vi "User_Event.vi"(0 "Event Data":T1, 11 "Error In":errorcluster, 13 "Enum":T2) -> (4 "Ref Out":refnum<user-event>, 15 "Error Out":errorcluster)   [LabVIEW 2020]
doc: "This VI is used to create, generate and destroy the user event."
uses:
  Typedef's/UserEvent_Operations.ctl
  Typedef's/Event_Data.ctl
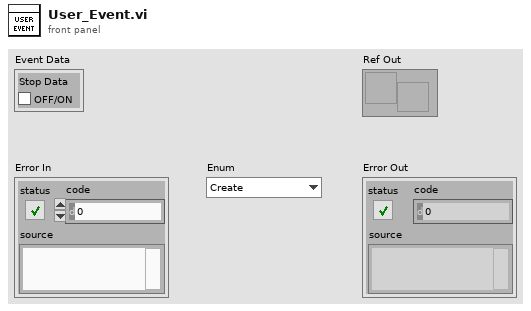
[diagram p1: front panel]
types:
  T1 = typedef "Event_Data.ctl" = cluster{"Stop Data":bool}
  T2 = typedef "UserEvent_Operations.ctl" = enum16{"Create", "Generate", "Get Ref", "Destroy"}
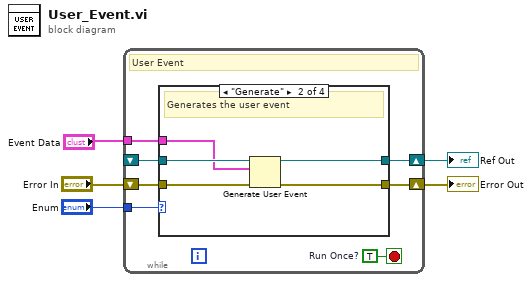
[diagram p0: block diagram]
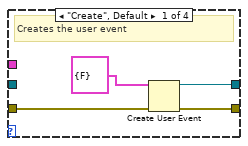
[diagram p2: hidden frame]
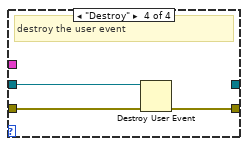
[diagram p4: hidden frame]
diagram:
  n1 = while {
    shift-right: [w8] -> w2
    shift-left: _ -> [w7]
    tunnel: "Enum" -> [w11]
    shift-right: [w9] -> w3
    shift-left: "Error In" -> [w10]
    tunnel: "Event Data" -> [w6]
    stop <- w12 stop-if-true
    w12 = TRUE  # Run Once?
    # "User Event"
    n2 = case shown="\"Generate\"" w11 {
      tunnel: [w15 w20 w23 w25] -> w9
      tunnel: w10 -> [w16 w21 w23 w26]
      tunnel: [w14 w18 w22 _] -> w8
      tunnel: w7 -> [_ w19 w22 w24]
      tunnel: w6 -> [_ w17 _ _]
      frame "Create", Default {
        # "Creates the user event"
        n3 = Create User Event(user event datatype=T1 {"Stop Data"=FALSE} ("Event Data"), error in=w16) -> (user event=w14:refnum<user-event>, error out=w15:errorcluster)
      }
      frame "Generate" {
        # "Generates the user event"
        n4 = Generate User Event(user event=w19, event data cluster=w17, error in=w21) -> (user event out=w18:refnum<user-event>, error out=w20:errorcluster)  [unwired: 1 in]
      }
      frame "Get Ref" {
        # "Do nothing. Just return the ref"
      }
      frame "Destroy" {
        # "destroy the user event"
        n5 = Destroy User Event(user event=w24, error in=w26) -> (error out=w25:errorcluster)
      }
    }
  }
  "Error Out" <- w3
  "Ref Out" <- w2
